vi "send.status.vi"(6 "iteration":i32, 8 "error in (no error)":errorcluster, 11 "ComicVine_manager in":refnum<class "ComicVine_manager.lvclass">) -> (0 "error out":errorcluster, 3 "ComicVine_manager out":refnum<class "ComicVine_manager.lvclass">)   [LabVIEW 2024, in "ComicVine_manager.lvclass"]
uses:
  ComicVine_manager.lvclass
  status--cluster.ctl
  ComicVine_manager.lvclass/ComicVine_manager.ctl
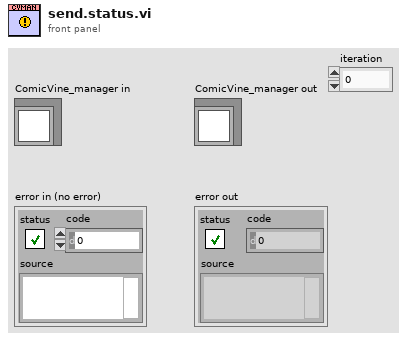
[diagram p1: front panel]
types:
  T1 = typedef "ComicVine_manager.lvclass/status--cluster.ctl" = cluster{"files in queue":i32, "in jail?":bool, "current state":string, "time left (s)":dbl, "iteration":i32, "error status":errorcluster, "log file":path}
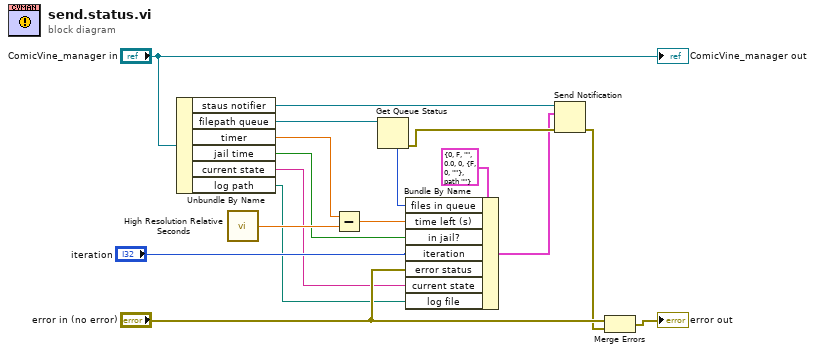
[diagram p0: block diagram]
diagram:
  n1 = Unbundle By Name("ComicVine_manager in") -> ("staus notifier"=w16:refnum<notifier>, "filepath queue"=w14:refnum<queue>, "timer"=w11:dbl, "jail time"=w8:bool, "current state"=w2:string, "log path"=w1:path)
  n2 = call <vilib>:"High Resolution Relative Seconds.vi"() -> ("relative seconds"=w10:dbl)
  n3 = Subtract(x=w11, y=w10) -> (x-y=w9:dbl)
  n4 = Get Queue Status(queue=w14) -> (error out=w12:errorcluster, # elements in queue=w13:i32)  [unwired: 2 in, 6 out]
  n5 = Bundle By Name(cluster=T1 {"files in queue"=0, "in jail?"=FALSE, "current state"="", "time left (s)"=0.0, "iteration"=0, "error status"={"status"=FALSE, "code"=0, "source"=""}, "log file"=path ""} ("status"), "files in queue"=w13, "time left (s)"=w9, "in jail?"=w8, "iteration"="iteration", "error status"="error in (no error)", "current state"=w2, "log file"=w1) -> (w7:T1)
  n6 = Send Notification(notification=w7, notifier=w16, error in (no error)=w12) -> (error out=w4:errorcluster)  [unwired: 1 out]
  n7 = Merge Errors("error in (no error)", w4) -> (→"error out":errorcluster)
  "ComicVine_manager out" <- "ComicVine_manager in"
